vi "Single Output Trigger Enable.vi"(8 "error in":errorcluster, 9 "State":i32(ring) items=["Active", "Inactive"], 10 "Trigger Output":i32(ring) items=["TTL0", "TTL1", "TTL2", "TTL3", "TTL4", "TTL5", "TTL6", "TTL7", "ECL0", "ECL1"], 11 "Instrument Handle In":i32) -> (0 "error out":errorcluster, 3 "Instrument Handle Out":i32)   [LabVIEW 8.6, in "ZTScopeM.lvlib"]
doc: "Configure the output state of the selected bus trigger line."
uses:
  ZTScopeM.lvlib
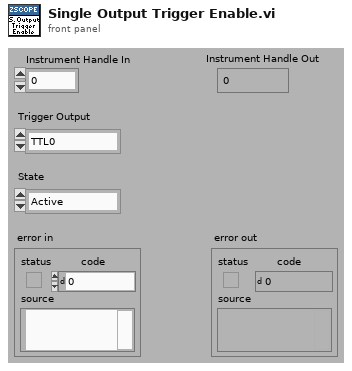
[diagram p1: front panel]
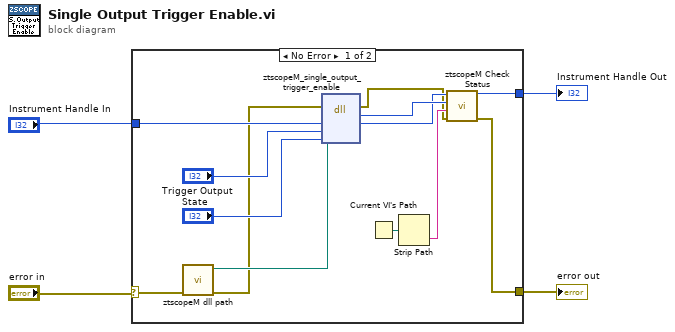
[diagram p0: block diagram]
diagram:
  n1 = case shown="No Error" "error in" {
    selector: "error in" -> [w9 w19]
    tunnel: [w12 w19] -> w3
    tunnel: [w13 w18] -> w2
    tunnel: "Instrument Handle In" -> [w7 w18]
    frame #0 {
      n2 = call "ztscopeM dll path.vi"("error in (no error)"=w9) -> ("error out"=w6:errorcluster, "<instrument>.dll path"=w8:path)  [unwired: 9 in]
      n3 = dll-call lib="C:/Program Files (x86)/National Instruments/LabVIEW 2013/instr.lib/ztscopem/ztscopeM.dll" fn="ztscopeM_single_output_trigger_enable"(path in=w8, error in=w6, "instrumentHandle"=w7, "triggerOutput"="Trigger Output", "state"="State") -> (error out=w5:errorcluster, w17:i32, "instrumentHandle"=w16:i32)  [unwired: 3 in, 1 out]
      n4 = Current VI's Path() -> (path=w15:path)
      n5 = Strip Path(path=w15) -> (name=w14:string)  [unwired: 1 out]
      n6 = call "ztscopeM Check Status.vi"("error in"=w5, "name of VI"=w14, "status (return code)"=w17, "instrument handle in"=w16) -> ("error out"=w12:errorcluster, "instrument handle out"=w13:i32)  [unwired: 2 out]
    }
    frame #1 {
    }
  }
  "Instrument Handle Out" <- w2
  "error out" <- w3
